vi "v3 ELEVADOR CHIDO.vi"(11 "Llama de Planta Baja":bool) -> ()   [LabVIEW 2018]
panel:
  out "Segundos de Prioridad":dbl
  in  "Abrir Puertas":bool
  out "Puerta Cerrada":bool
  out "Puerta abierta":bool
  out "Segundos de Inactividad":dbl
  in  "Ir a B 2":bool
  out "Piso actual":bool[](array[boolean])
  in  "Piso 2":bool
  in  "Piso 1":bool
  in  "Planta Baja":bool
  in  "Llama de Piso 2":bool
  in  "Llama de Piso 1":bool
  in  "Alarma":bool
  # "Límite de inactividad:\n1 minuto para regresar\na Planta Baja"
  # "PB"
  # "Para lograr detectar la prioridad\n debe ser dentro de 3 segundos"
  # "P1"
  # "P2"
  # "Pulsadores Externos"
  # "Pulsadores Internos"
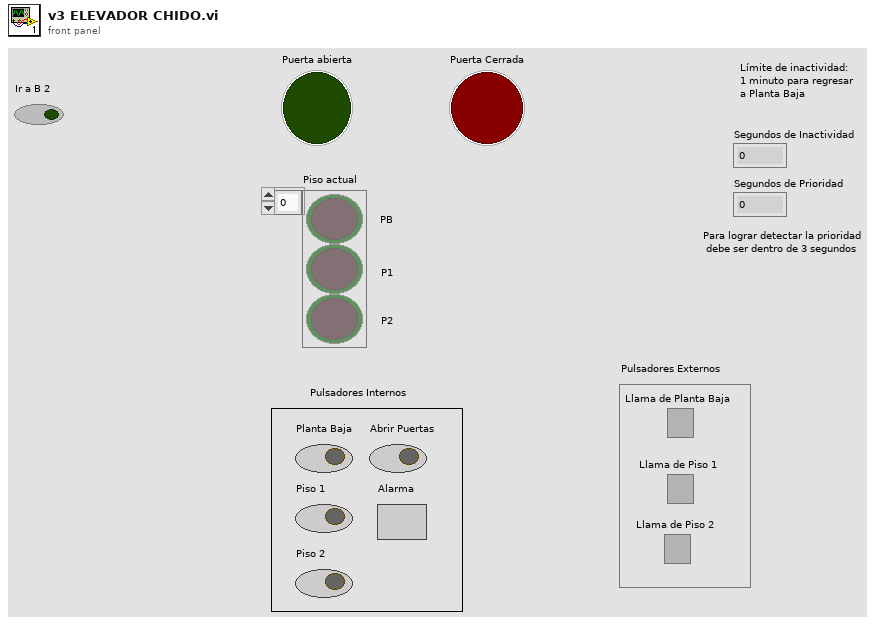
[diagram p1: front panel]
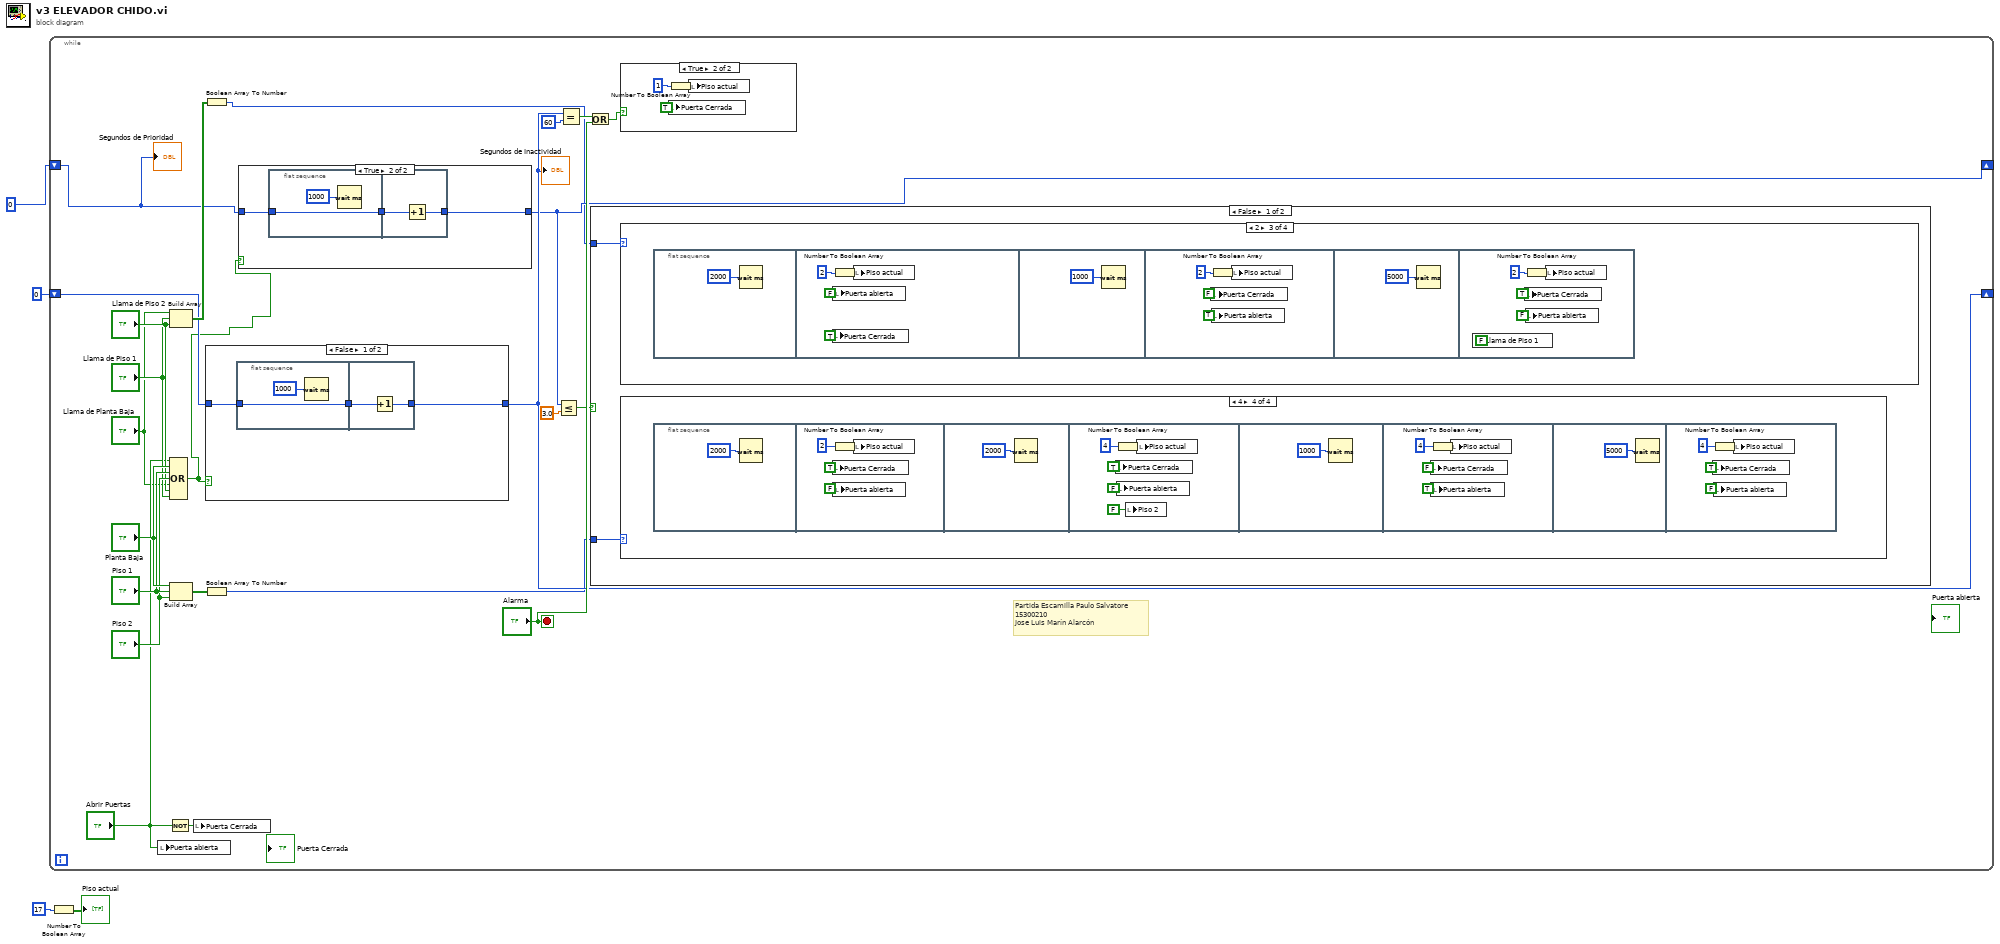
[diagram p0: block diagram]
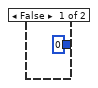
[diagram p2: hidden frame]
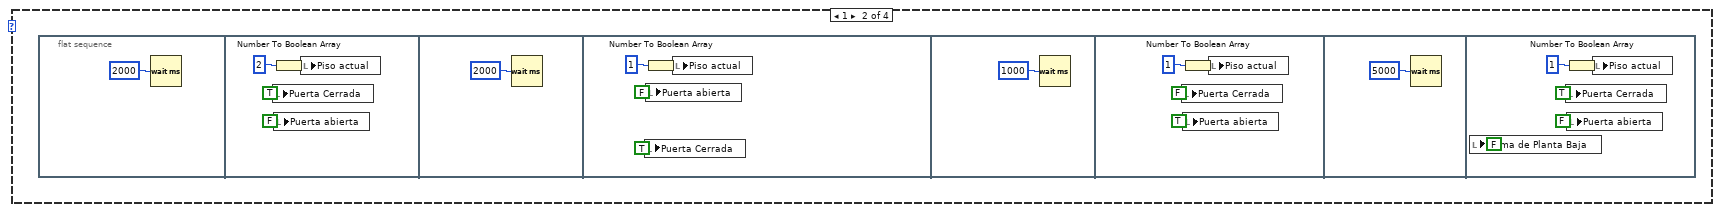
[diagram p4: hidden frame]
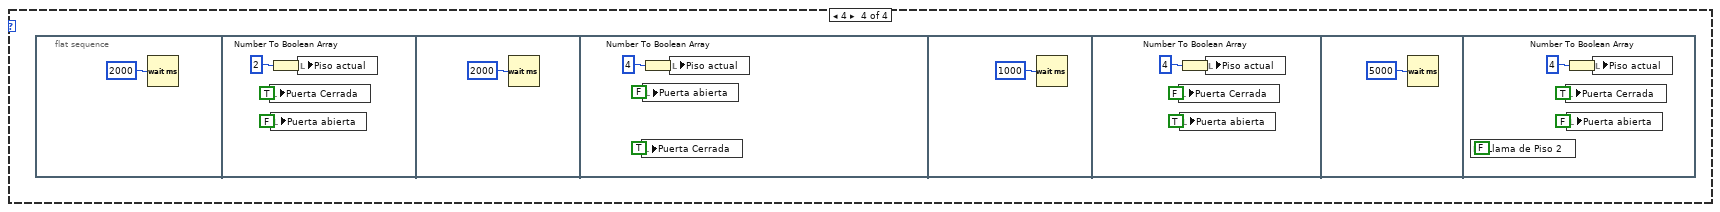
[diagram p5: hidden frame]
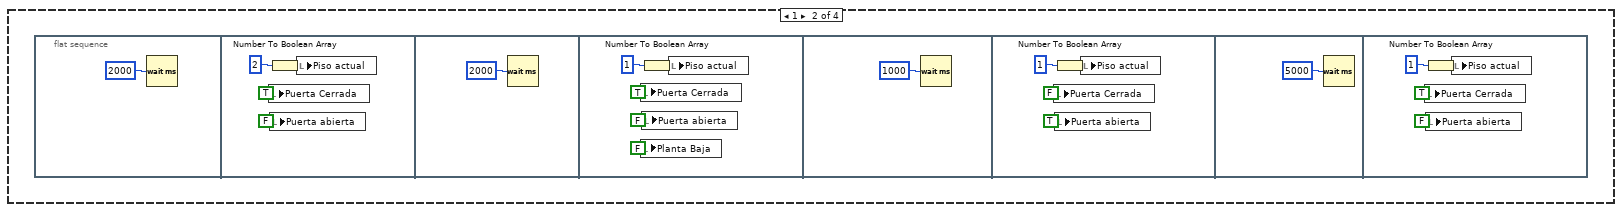
[diagram p7: hidden frame]
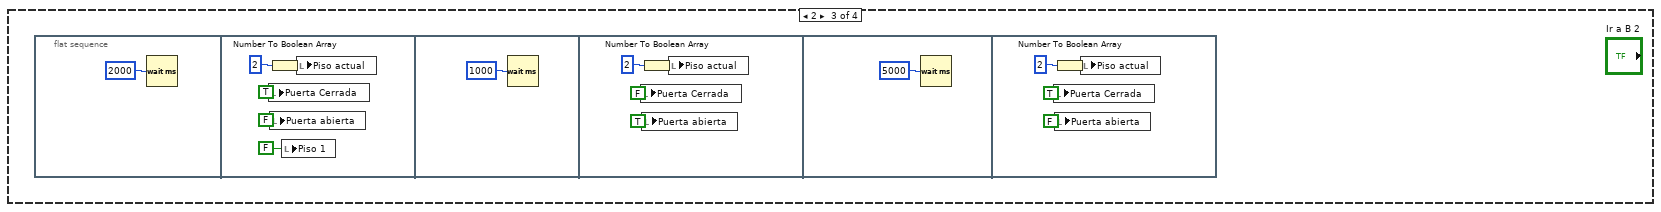
[diagram p8: hidden frame]
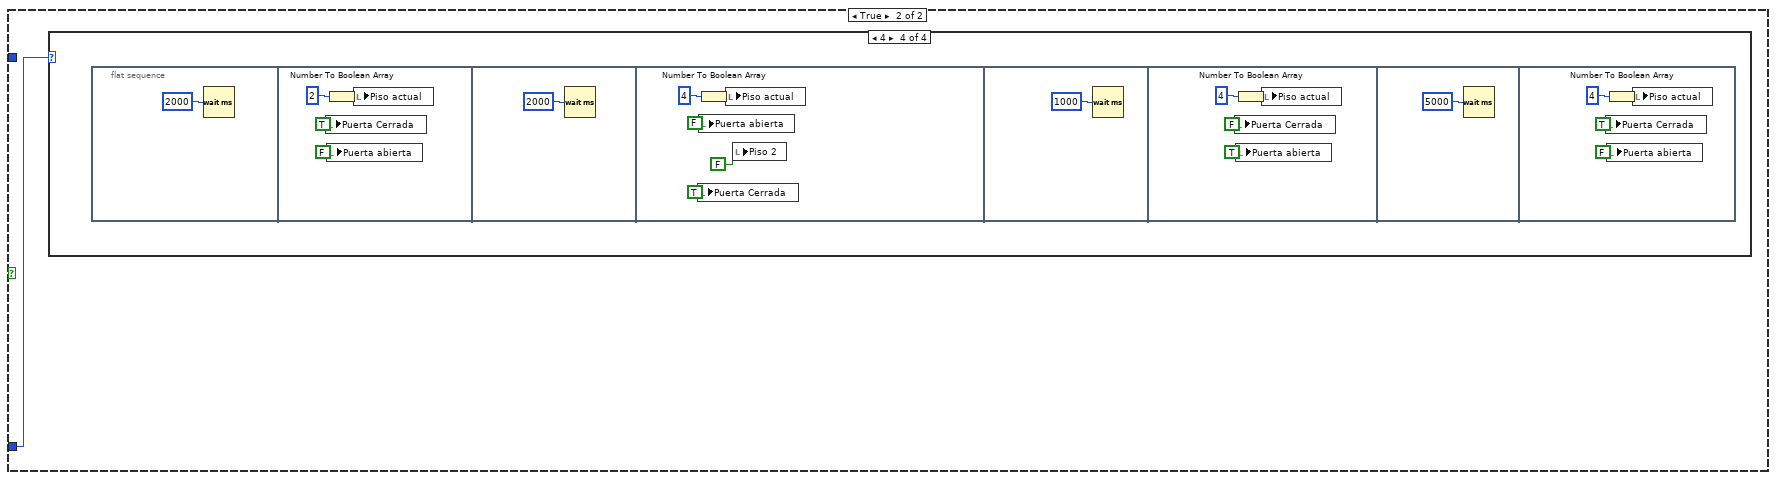
[diagram p9: hidden frame]
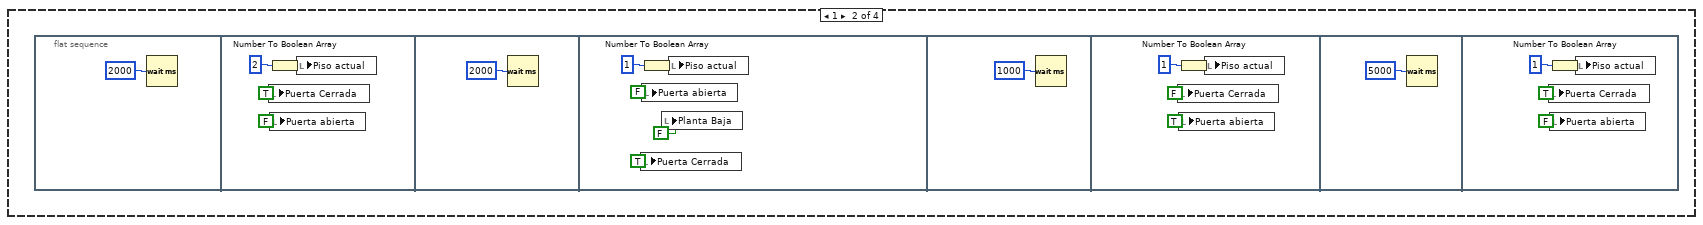
[diagram p11: hidden frame]
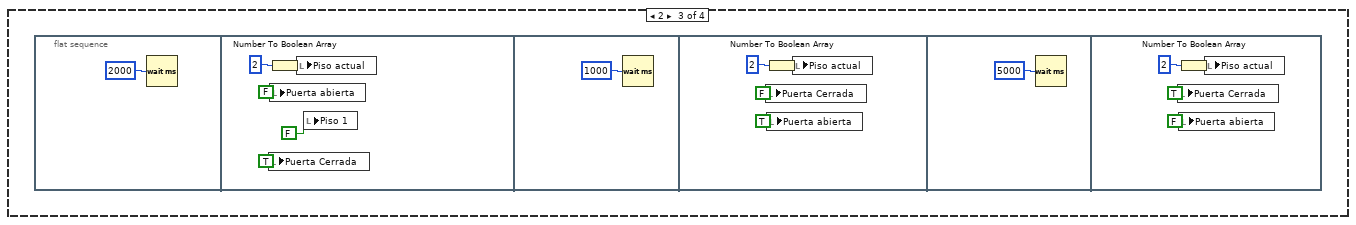
[diagram p12: hidden frame]
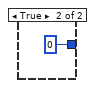
[diagram p14: hidden frame]
diagram:
  n1 = while {
    shift-right: [w12] -> _
    shift-left: 0 -> [w20]
    shift-right: [w7] -> _
    shift-left: 0 -> [w9]
    stop <- "Alarma" stop-if-true
    # "Partida Escamilla Paulo Salvatore\n15300210\nJose Luis Marín Alarcón"
    n2 = local write "Puerta abierta"("Abrir Puertas") -> ()
    n3 = Not(x="Abrir Puertas") -> (.not. x?=w15:bool)
    n4 = Build Array("Llama de Planta Baja", "Llama de Piso 1", "Llama de Piso 2") -> (w27:bool[])
    n5 = Build Array("Planta Baja", "Piso 1", "Piso 2") -> (w26:bool[])
    n6 = Compound Arithmetic op=OR("Abrir Puertas", "Planta Baja", "Piso 1", "Piso 2", "Llama de Planta Baja", "Llama de Piso 2", "Llama de Piso 1") -> (w8:bool)
    n7 = local write "Puerta Cerrada"(w15) -> ()
    n8 = Boolean Array To Number(Boolean array=w27) -> (number=w5:u32)
    n9 = Boolean Array To Number(Boolean array=w26) -> (number=w10:u32)
    n10 = case shown="False" w8 {
      tunnel: w20 -> [w218 _]
      tunnel: [w216 0] -> w12
      frame False {
        n11 = flat-sequence {
          tunnel: w218 -> [w219]
          tunnel: [w219] -> w217
          tunnel: w217 -> [w222]
          tunnel: [w221] -> w216
          frame #0 {
            n12 = Wait (ms)(milliseconds to wait=u32 1000) -> ()  [unwired: 1 out]
          }
          frame #1 {
            n13 = Increment(x=w222) -> (x+1=w221:i32)
          }
        }
      }
      frame True {
      }
    }
    "Segundos de Inactividad" <- w12
    n14 = case shown="True" w8 {
      tunnel: w9 -> [_ w31]
      tunnel: [0 w29] -> w7
      frame False {
      }
      frame True {
        n15 = flat-sequence {
          tunnel: w31 -> [w32]
          tunnel: [w32] -> w30
          tunnel: w30 -> [w35]
          tunnel: [w34] -> w29
          frame #0 {
            n16 = Wait (ms)(milliseconds to wait=u32 1000) -> ()  [unwired: 1 out]
          }
          frame #1 {
            n17 = Increment(x=w35) -> (x+1=w34:i32)
          }
        }
      }
    }
    n18 = Less Or Equal?(x=w7, y=3.0) -> (x <= y?=w11:bool)
    n19 = Equal?(x=w12, y=60) -> (x = y?=w18:bool)
    n20 = Or(x=w18, y="Alarma") -> (x .or. y?=w17:bool)
    n21 = case shown="False" w11 {
      tunnel: w5 -> [w36 _]
      tunnel: w10 -> [w37 w154]
      frame False {
        n22 = case shown="2" w36 {
          frame 0, Default {
          }
          frame 1 {
            n23 = flat-sequence {
              frame #0 {
                n24 = Wait (ms)(milliseconds to wait=u32 2000) -> ()  [unwired: 1 out]
              }
              frame #1 {
                n25 = local write "Puerta Cerrada"(TRUE) -> ()
                n26 = Number To Boolean Array(number=2) -> (Boolean array=w41:bool[])
                n27 = local write "Puerta abierta"(FALSE) -> ()
                n28 = local write "Piso actual"(w41) -> ()
              }
              frame #2 {
                n29 = Wait (ms)(milliseconds to wait=u32 2000) -> ()  [unwired: 1 out]
              }
              frame #3 {
                n30 = local write "Puerta Cerrada"(TRUE) -> ()
                n31 = Number To Boolean Array(number=1) -> (Boolean array=w46:bool[])
                n32 = local write "Puerta abierta"(FALSE) -> ()
                n33 = local write "Piso actual"(w46) -> ()
              }
              frame #4 {
                n34 = Wait (ms)(milliseconds to wait=u32 1000) -> ()  [unwired: 1 out]
              }
              frame #5 {
                n35 = local write "Puerta Cerrada"(FALSE) -> ()
                n36 = Number To Boolean Array(number=1) -> (Boolean array=w52:bool[])
                n37 = local write "Puerta abierta"(TRUE) -> ()
                n38 = local write "Piso actual"(w52) -> ()
              }
              frame #6 {
                n39 = Wait (ms)(milliseconds to wait=u32 5000) -> ()  [unwired: 1 out]
              }
              frame #7 {
                n40 = local write "Llama de Planta Baja"(FALSE) -> ()
                n41 = local write "Puerta Cerrada"(TRUE) -> ()
                n42 = Number To Boolean Array(number=1) -> (Boolean array=w57:bool[])
                n43 = local write "Puerta abierta"(FALSE) -> ()
                n44 = local write "Piso actual"(w57) -> ()
              }
            }
          }
          frame 2 {
            n45 = flat-sequence {
              frame #0 {
                n46 = Wait (ms)(milliseconds to wait=u32 2000) -> ()  [unwired: 1 out]
              }
              frame #1 {
                n47 = local write "Puerta Cerrada"(TRUE) -> ()
                n48 = Number To Boolean Array(number=2) -> (Boolean array=w62:bool[])
                n49 = local write "Puerta abierta"(FALSE) -> ()
                n50 = local write "Piso actual"(w62) -> ()
              }
              frame #2 {
                n51 = Wait (ms)(milliseconds to wait=u32 1000) -> ()  [unwired: 1 out]
              }
              frame #3 {
                n52 = local write "Puerta Cerrada"(FALSE) -> ()
                n53 = Number To Boolean Array(number=2) -> (Boolean array=w67:bool[])
                n54 = local write "Puerta abierta"(TRUE) -> ()
                n55 = local write "Piso actual"(w67) -> ()
              }
              frame #4 {
                n56 = Wait (ms)(milliseconds to wait=u32 5000) -> ()  [unwired: 1 out]
              }
              frame #5 {
                n57 = local write "Llama de Piso 1"(FALSE) -> ()
                n58 = local write "Puerta Cerrada"(TRUE) -> ()
                n59 = Number To Boolean Array(number=2) -> (Boolean array=w73:bool[])
                n60 = local write "Puerta abierta"(FALSE) -> ()
                n61 = local write "Piso actual"(w73) -> ()
              }
            }
          }
          frame 4 {
            n62 = flat-sequence {
              frame #0 {
                n63 = Wait (ms)(milliseconds to wait=u32 2000) -> ()  [unwired: 1 out]
              }
              frame #1 {
                n64 = local write "Puerta Cerrada"(TRUE) -> ()
                n65 = Number To Boolean Array(number=2) -> (Boolean array=w78:bool[])
                n66 = local write "Puerta abierta"(FALSE) -> ()
                n67 = local write "Piso actual"(w78) -> ()
              }
              frame #2 {
                n68 = Wait (ms)(milliseconds to wait=u32 2000) -> ()  [unwired: 1 out]
              }
              frame #3 {
                n69 = local write "Puerta Cerrada"(TRUE) -> ()
                n70 = Number To Boolean Array(number=4) -> (Boolean array=w83:bool[])
                n71 = local write "Puerta abierta"(FALSE) -> ()
                n72 = local write "Piso actual"(w83) -> ()
              }
              frame #4 {
                n73 = Wait (ms)(milliseconds to wait=u32 1000) -> ()  [unwired: 1 out]
              }
              frame #5 {
                n74 = local write "Puerta Cerrada"(FALSE) -> ()
                n75 = Number To Boolean Array(number=4) -> (Boolean array=w88:bool[])
                n76 = local write "Puerta abierta"(TRUE) -> ()
                n77 = local write "Piso actual"(w88) -> ()
              }
              frame #6 {
                n78 = Wait (ms)(milliseconds to wait=u32 5000) -> ()  [unwired: 1 out]
              }
              frame #7 {
                n79 = local write "Llama de Piso 2"(FALSE) -> ()
                n80 = local write "Puerta Cerrada"(TRUE) -> ()
                n81 = Number To Boolean Array(number=4) -> (Boolean array=w94:bool[])
                n82 = local write "Puerta abierta"(FALSE) -> ()
                n83 = local write "Piso actual"(w94) -> ()
              }
            }
          }
        }
        n84 = case shown="4" w37 {
          frame 0, Default {
          }
          frame 1 {
            n85 = flat-sequence {
              frame #0 {
                n86 = Wait (ms)(milliseconds to wait=u32 2000) -> ()  [unwired: 1 out]
              }
              frame #1 {
                n87 = local write "Puerta Cerrada"(TRUE) -> ()
                n88 = Number To Boolean Array(number=2) -> (Boolean array=w99:bool[])
                n89 = local write "Puerta abierta"(FALSE) -> ()
                n90 = local write "Piso actual"(w99) -> ()
              }
              frame #2 {
                n91 = Wait (ms)(milliseconds to wait=u32 2000) -> ()  [unwired: 1 out]
              }
              frame #3 {
                n92 = local write "Puerta Cerrada"(TRUE) -> ()
                n93 = local write "Planta Baja"(FALSE) -> ()
                n94 = Number To Boolean Array(number=1) -> (Boolean array=w105:bool[])
                n95 = local write "Puerta abierta"(FALSE) -> ()
                n96 = local write "Piso actual"(w105) -> ()
              }
              frame #4 {
                n97 = Wait (ms)(milliseconds to wait=u32 1000) -> ()  [unwired: 1 out]
              }
              frame #5 {
                n98 = local write "Puerta Cerrada"(FALSE) -> ()
                n99 = Number To Boolean Array(number=1) -> (Boolean array=w110:bool[])
                n100 = local write "Puerta abierta"(TRUE) -> ()
                n101 = local write "Piso actual"(w110) -> ()
              }
              frame #6 {
                n102 = Wait (ms)(milliseconds to wait=u32 5000) -> ()  [unwired: 1 out]
              }
              frame #7 {
                n103 = local write "Puerta Cerrada"(TRUE) -> ()
                n104 = Number To Boolean Array(number=1) -> (Boolean array=w115:bool[])
                n105 = local write "Puerta abierta"(FALSE) -> ()
                n106 = local write "Piso actual"(w115) -> ()
              }
            }
          }
          frame 2 {
            n107 = flat-sequence {
              frame #0 {
                n108 = Wait (ms)(milliseconds to wait=u32 2000) -> ()  [unwired: 1 out]
              }
              frame #1 {
                n109 = local write "Puerta Cerrada"(TRUE) -> ()
                n110 = Number To Boolean Array(number=2) -> (Boolean array=w121:bool[])
                n111 = local write "Puerta abierta"(FALSE) -> ()
                n112 = local write "Piso 1"(FALSE) -> ()
                n113 = local write "Piso actual"(w121) -> ()
              }
              frame #2 {
                n114 = Wait (ms)(milliseconds to wait=u32 1000) -> ()  [unwired: 1 out]
              }
              frame #3 {
                n115 = local write "Puerta Cerrada"(FALSE) -> ()
                n116 = Number To Boolean Array(number=2) -> (Boolean array=w126:bool[])
                n117 = local write "Puerta abierta"(TRUE) -> ()
                n118 = local write "Piso actual"(w126) -> ()
              }
              frame #4 {
                n119 = Wait (ms)(milliseconds to wait=u32 5000) -> ()  [unwired: 1 out]
              }
              frame #5 {
                n120 = local write "Puerta Cerrada"(TRUE) -> ()
                n121 = Number To Boolean Array(number=2) -> (Boolean array=w131:bool[])
                n122 = local write "Puerta abierta"(FALSE) -> ()
                n123 = local write "Piso actual"(w131) -> ()
              }
            }
          }
          frame 4 {
            n124 = flat-sequence {
              frame #0 {
                n125 = Wait (ms)(milliseconds to wait=u32 2000) -> ()  [unwired: 1 out]
              }
              frame #1 {
                n126 = local write "Puerta Cerrada"(TRUE) -> ()
                n127 = Number To Boolean Array(number=2) -> (Boolean array=w136:bool[])
                n128 = local write "Puerta abierta"(FALSE) -> ()
                n129 = local write "Piso actual"(w136) -> ()
              }
              frame #2 {
                n130 = Wait (ms)(milliseconds to wait=u32 2000) -> ()  [unwired: 1 out]
              }
              frame #3 {
                n131 = local write "Puerta Cerrada"(TRUE) -> ()
                n132 = Number To Boolean Array(number=4) -> (Boolean array=w142:bool[])
                n133 = local write "Puerta abierta"(FALSE) -> ()
                n134 = local write "Piso 2"(FALSE) -> ()
                n135 = local write "Piso actual"(w142) -> ()
              }
              frame #4 {
                n136 = Wait (ms)(milliseconds to wait=u32 1000) -> ()  [unwired: 1 out]
              }
              frame #5 {
                n137 = local write "Puerta Cerrada"(FALSE) -> ()
                n138 = Number To Boolean Array(number=4) -> (Boolean array=w147:bool[])
                n139 = local write "Puerta abierta"(TRUE) -> ()
                n140 = local write "Piso actual"(w147) -> ()
              }
              frame #6 {
                n141 = Wait (ms)(milliseconds to wait=u32 5000) -> ()  [unwired: 1 out]
              }
              frame #7 {
                n142 = local write "Puerta Cerrada"(TRUE) -> ()
                n143 = Number To Boolean Array(number=4) -> (Boolean array=w152:bool[])
                n144 = local write "Puerta abierta"(FALSE) -> ()
                n145 = local write "Piso actual"(w152) -> ()
              }
            }
          }
        }
      }
      frame True {
        n146 = case shown="4" w154 {
          frame 0, Default {
          }
          frame 1 {
            n147 = flat-sequence {
              frame #0 {
                n148 = Wait (ms)(milliseconds to wait=u32 2000) -> ()  [unwired: 1 out]
              }
              frame #1 {
                n149 = local write "Puerta Cerrada"(TRUE) -> ()
                n150 = Number To Boolean Array(number=2) -> (Boolean array=w158:bool[])
                n151 = local write "Puerta abierta"(FALSE) -> ()
                n152 = local write "Piso actual"(w158) -> ()
              }
              frame #2 {
                n153 = Wait (ms)(milliseconds to wait=u32 2000) -> ()  [unwired: 1 out]
              }
              frame #3 {
                n154 = local write "Puerta Cerrada"(TRUE) -> ()
                n155 = Number To Boolean Array(number=1) -> (Boolean array=w164:bool[])
                n156 = local write "Puerta abierta"(FALSE) -> ()
                n157 = local write "Planta Baja"(FALSE) -> ()
                n158 = local write "Piso actual"(w164) -> ()
              }
              frame #4 {
                n159 = Wait (ms)(milliseconds to wait=u32 1000) -> ()  [unwired: 1 out]
              }
              frame #5 {
                n160 = local write "Puerta Cerrada"(FALSE) -> ()
                n161 = Number To Boolean Array(number=1) -> (Boolean array=w170:bool[])
                n162 = local write "Puerta abierta"(TRUE) -> ()
                n163 = local write "Piso actual"(w170) -> ()
              }
              frame #6 {
                n164 = Wait (ms)(milliseconds to wait=u32 5000) -> ()  [unwired: 1 out]
              }
              frame #7 {
                n165 = local write "Puerta Cerrada"(TRUE) -> ()
                n166 = Number To Boolean Array(number=1) -> (Boolean array=w174:bool[])
                n167 = local write "Puerta abierta"(FALSE) -> ()
                n168 = local write "Piso actual"(w174) -> ()
              }
            }
          }
          frame 2 {
            n169 = flat-sequence {
              frame #0 {
                n170 = Wait (ms)(milliseconds to wait=u32 2000) -> ()  [unwired: 1 out]
              }
              frame #1 {
                n171 = local write "Puerta Cerrada"(TRUE) -> ()
                n172 = Number To Boolean Array(number=2) -> (Boolean array=w180:bool[])
                n173 = local write "Puerta abierta"(FALSE) -> ()
                n174 = local write "Piso actual"(w180) -> ()
                n175 = local write "Piso 1"(FALSE) -> ()
              }
              frame #2 {
                n176 = Wait (ms)(milliseconds to wait=u32 1000) -> ()  [unwired: 1 out]
              }
              frame #3 {
                n177 = local write "Puerta Cerrada"(FALSE) -> ()
                n178 = Number To Boolean Array(number=2) -> (Boolean array=w185:bool[])
                n179 = local write "Puerta abierta"(TRUE) -> ()
                n180 = local write "Piso actual"(w185) -> ()
              }
              frame #4 {
                n181 = Wait (ms)(milliseconds to wait=u32 5000) -> ()  [unwired: 1 out]
              }
              frame #5 {
                n182 = local write "Puerta Cerrada"(TRUE) -> ()
                n183 = Number To Boolean Array(number=2) -> (Boolean array=w190:bool[])
                n184 = local write "Puerta abierta"(FALSE) -> ()
                n185 = local write "Piso actual"(w190) -> ()
              }
            }
          }
          frame 4 {
            n186 = flat-sequence {
              frame #0 {
                n187 = Wait (ms)(milliseconds to wait=u32 2000) -> ()  [unwired: 1 out]
              }
              frame #1 {
                n188 = local write "Puerta Cerrada"(TRUE) -> ()
                n189 = Number To Boolean Array(number=2) -> (Boolean array=w195:bool[])
                n190 = local write "Puerta abierta"(FALSE) -> ()
                n191 = local write "Piso actual"(w195) -> ()
              }
              frame #2 {
                n192 = Wait (ms)(milliseconds to wait=u32 2000) -> ()  [unwired: 1 out]
              }
              frame #3 {
                n193 = local write "Puerta Cerrada"(TRUE) -> ()
                n194 = Number To Boolean Array(number=4) -> (Boolean array=w201:bool[])
                n195 = local write "Puerta abierta"(FALSE) -> ()
                n196 = local write "Piso actual"(w201) -> ()
                n197 = local write "Piso 2"(FALSE) -> ()
              }
              frame #4 {
                n198 = Wait (ms)(milliseconds to wait=u32 1000) -> ()  [unwired: 1 out]
              }
              frame #5 {
                n199 = local write "Puerta Cerrada"(FALSE) -> ()
                n200 = Number To Boolean Array(number=4) -> (Boolean array=w206:bool[])
                n201 = local write "Puerta abierta"(TRUE) -> ()
                n202 = local write "Piso actual"(w206) -> ()
              }
              frame #6 {
                n203 = Wait (ms)(milliseconds to wait=u32 5000) -> ()  [unwired: 1 out]
              }
              frame #7 {
                n204 = local write "Puerta Cerrada"(TRUE) -> ()
                n205 = Number To Boolean Array(number=4) -> (Boolean array=w211:bool[])
                n206 = local write "Puerta abierta"(FALSE) -> ()
                n207 = local write "Piso actual"(w211) -> ()
              }
            }
          }
        }
      }
    }
    n208 = case shown="True" w17 {
      frame False {
      }
      frame True {
        n209 = local write "Puerta Cerrada"(TRUE) -> ()
        n210 = Number To Boolean Array(number=1) -> (Boolean array=w215:bool[])
        n211 = local write "Piso actual"(w215) -> ()
      }
    }
    "Segundos de Prioridad" <- w9
  }
  n212 = Number To Boolean Array(number=u32 17) -> (Boolean array=→"Piso actual":bool[])
